vi "Finish.vi"   [LabVIEW 2015]
doc: "This VI is called just before exiting. It is expected to close I/O refnum, save collected data, etc."
uses:
  <vilib>/Rock Robotics/WPI/Utilities/WPI_GetSetVariantRefNum.vi
types:
  T1 = typedef "WPI_DigitalInputDevRef.ctl" = cluster{"DevStatus":errorcluster, "DIO Channel":T2}
  T2 = typedef "FPGA_DIOChannel.ctl" = enum8{"DIO 0", "DIO 1", "DIO 2", "DIO 3", "DIO 4", "DIO 5", "DIO 6", "DIO 7", "DIO 8", "DIO 9", "DIO MXP 0", "DIO MXP 1", "DIO MXP 2", "DIO MXP 3", "DIO MXP 4", "DIO MXP 5", "DIO MXP 6", "DIO MXP 7", "DIO MXP 8", "DIO MXP 9", "DIO MXP 10", "DIO MXP 11", "DIO MXP 12", "DIO MXP 13", "DIO MXP 14", "DIO MXP 15", "Invalid"}
  T3 = typedef "WPI_AccelerometerDevRef.ctl" = cluster{"DevStatus":errorcluster, "Scaling":T4, "Analog Channels":T5, "I2C Bus":T7, "SPI Bus":T8, "Accel Range":T9, "ADXL Axes":T10, "Handle":i32, "Device Address":u8, "Accel Type":enum16{"Analog", "ADXL345 I2C", "ADXL345 SPI", "Internal", "ADXL362 SPI"}}
  T4 = typedef "WPI_AccelerometerScaling.ctl" = cluster{"Gain (VoltsPerG)":dbl, "Center Voltage":dbl}
  T5 = typedef "WPI_AccelerometerAnalogChannels.ctl" = cluster{"X-Axis":T6, "Y-Axis":T6, "Z-Axis":T6}
  T6 = typedef "FPGA_AIChannel.ctl" = enum8{"AI 0", "AI 1", "AI 2", "AI 3", "AI MXP 0", "AI MXP 1", "AI MXP 2", "AI MXP 3", "Invalid"}
  T7 = typedef "i2c_bus.ctl" = enum16{"I2C On-Board", "I2C MXP", "Invalid"}
  T8 = typedef "spi_bus.ctl" = enum16{"SPI On-Board, CS0", "SPI On-Board, CS1", "SPI On-Board, CS2", "SPI On-Board, CS3", "SPI MXP", "Invalid"}
  T9 = typedef "ADXL345 Range.ctl" = u8
  T10 = typedef "WPI_AccelerometerADXL345 Axes.ctl" = cluster{"X-Axis":bool, "Y-Axis":bool, "Z-Axis":bool}
  T11 = typedef "WPI_SolenoidDevRef.ctl" = cluster{"DevStatus":errorcluster, "Pneumatics Control Module":u8, "Forward Solenoid Channel":T12, "Reverse Solenoid Channel":T12}
  T12 = typedef "WPI_SolenoidChannel.ctl" = enum8{"Solenoid 0", "Solenoid 1", "Solenoid 2", "Solenoid 3", "Solenoid 4", "Solenoid 5", "Solenoid 6", "Solenoid 7", "Invalid"}
  T13 = typedef "WPI_ServoDeviceRef.ctl" = cluster{"DeviceStatus":errorcluster, "PWM Channel":T14, "DeadBand":T15}
  T14 = typedef "FPGA_DIOPWMChannel.ctl" = enum8{"PWM 0", "PWM 1", "PWM 2", "PWM 3", "PWM 4", "PWM 5", "PWM 6", "PWM 7", "PWM 8", "PWM 9", "PWM MXP 0", "PWM MXP 1", "PWM MXP 2", "PWM MXP 3", "PWM MXP 4", "PWM MXP 5", "PWM MXP 6", "PWM MXP 7", "PWM MXP 8", "PWM MXP 9", "Invalid"}
  T15 = typedef "WPI_PWMDeadband.ctl" = cluster{"Name":string, "maxPositivePwm":i32, "minPositivePwm":i32, "centerPwm":i32, "maxNegativePwm":i32, "minNegativePwm":i32, "angularRange":u16}
  T16 = typedef "WPI_MotorControlDeviceRef.ctl" = cluster{"DeviceStatus":errorcluster, "Type":T17, "PWM":cluster{"PWM Channel":T14, "DeadBand":T15}, "CAN":cluster{"Device Number":u8, "Control Mode":T18, "Semaphore":T19, "Max Vout":dbl, "TalonSRX Control Mode":T20}, "Invert":bool}
  T17 = typedef "WPI_MotorControlType.ctl" = enum16{"PWM", "CAN", "CANTalonSRX"}
  T18 = typedef "WPI_CANJaguar_ControlMode.ctl" = enum8{"Percent VBus", "Current", "Speed", "Position", "Voltage"}
  T19 = typedef "Semaphore RefNum" = refnum<k1>
  T20 = typedef "WPI_CANTalonSRX_APIControlMode.ctl" = enum8{"Percent VBus", "Speed", "Position", "Slave", "Unchanged / Invalid", "Voltage Compensation", "Current", "Motion Profile"}
  T21 = typedef "WPI_JoystickDevRef.ctl" = cluster{"Device":T22}
  T22 = typedef "WPI_JoystickDeviceEnum.ctl" = enum16{"USB 0", "USB 1", "USB 2", "USB 3", "USB 4", "USB 5"}
  T23 = typedef "WPI_RobotDriveDevRef.ctl" = cluster{"DevStatus":errorcluster, "Motors[]":T16[], "Square Inputs":bool, "Max Output":dbl}
  T24 = typedef "WPI_GyroDevRef.ctl" = cluster{"DevStatus":errorcluster, "Analog Channel":T6, "Offset":dbl, "Gain (VoltsPerDegree/Second)":dbl, "Gyro Type":enum16{"Analog", "XRS450"}, "Handle":i32, "SPI Bus":T8, "Device Found":bool, "Sample Rate":dbl, "Calibrate On Open":bool}
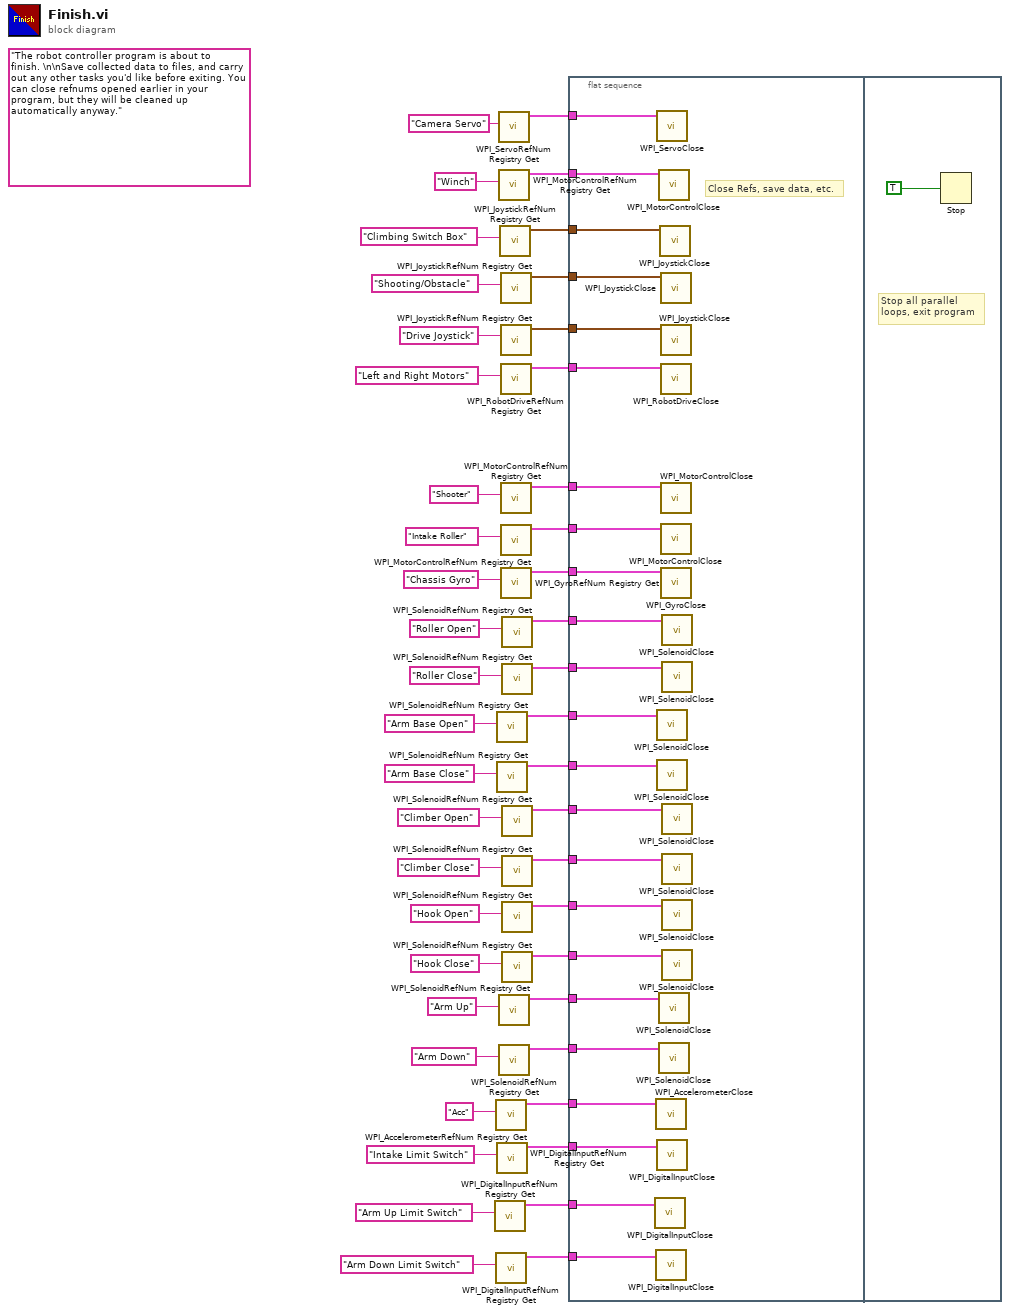
[diagram p0: block diagram]
diagram:
  (unwired) "The robot controller program is about to finish. \n\nSave collected data to files, and carry out any other tasks you'd like before exiting. You can close refnums opened earlier in your program, but they will be cleaned up automatically anyway."
  n1 = call <vilib>:"WPI_DigitalInputRefNum Registry Get.vi"("refnum name"="Arm Up Limit Switch") -> ("DigitalInputDevRef"=w15:T1)  [unwired: 9 in, 1 out]
  n2 = call <vilib>:"WPI_AccelerometerRefNum Registry Get.vi"("refnum name"="Acc") -> ("AccelerometerDevRef"=w36:T3)  [unwired: 9 in, 1 out]
  n3 = call <vilib>:"WPI_DigitalInputRefNum Registry Get.vi"("refnum name"="Arm Down Limit Switch") -> ("DigitalInputDevRef"=w14:T1)  [unwired: 9 in, 1 out]
  n4 = call <vilib>:"WPI_SolenoidRefNum Registry Get.vi"("refnum name"="Arm Base Open") -> ("SolenoidDevRef"=w12:T11)  [unwired: 9 in, 1 out]
  n5 = call <vilib>:"WPI_SolenoidRefNum Registry Get.vi"("refnum name"="Arm Base Close") -> ("SolenoidDevRef"=w9:T11)  [unwired: 9 in, 1 out]
  n6 = call <vilib>:"WPI_DigitalInputRefNum Registry Get.vi"("refnum name"="Intake Limit Switch") -> ("DigitalInputDevRef"=w38:T1)  [unwired: 9 in, 1 out]
  n7 = call <vilib>:"WPI_ServoRefNum Registry Get.vi"("refnum name"="Camera Servo") -> ("ServoDeviceRef"=w2:T13)  [unwired: 9 in, 1 out]
  n8 = call <vilib>:"WPI_MotorControlRefNum Registry Get.vi"("refnum name"="Winch") -> ("MotorControlDevRef"=w17:T16)  [unwired: 9 in, 1 out]
  n9 = call <vilib>:"WPI_SolenoidRefNum Registry Get.vi"("refnum name"="Arm Up") -> ("SolenoidDevRef"=w5:T11)  [unwired: 9 in, 1 out]
  n10 = call <vilib>:"WPI_SolenoidRefNum Registry Get.vi"("refnum name"="Arm Down") -> ("SolenoidDevRef"=w8:T11)  [unwired: 9 in, 1 out]
  n11 = call <vilib>:"WPI_JoystickRefNum Registry Get.vi"("refnum name"="Climbing Switch Box") -> ("JoystickDevRef"=w4:T21)  [unwired: 1 in, 9 out]
  n12 = call <vilib>:"WPI_JoystickRefNum Registry Get.vi"("refnum name"="Shooting/Obstacle") -> ("JoystickDevRef"=w43:T21)  [unwired: 1 in, 9 out]
  n13 = call <vilib>:"WPI_JoystickRefNum Registry Get.vi"("refnum name"="Drive Joystick") -> ("JoystickDevRef"=w32:T21)  [unwired: 1 in, 9 out]
  n14 = call <vilib>:"WPI_RobotDriveRefNum Registry Get.vi"("refnum name"="Left and Right Motors") -> ("RobotDriveDevRef"=w44:T23)  [unwired: 1 in, 9 out]
  n15 = call <vilib>:"WPI_MotorControlRefNum Registry Get.vi"("refnum name"="Shooter") -> ("MotorControlDevRef"=w42:T16)  [unwired: 9 in, 1 out]
  n16 = call <vilib>:"WPI_MotorControlRefNum Registry Get.vi"("refnum name"="Intake Roller") -> ("MotorControlDevRef"=w33:T16)  [unwired: 9 in, 1 out]
  n17 = call <vilib>:"WPI_GyroRefNum Registry Get.vi"("refnum name"="Chassis Gyro") -> ("GyroDevRef"=w40:T24)  [unwired: 9 in, 1 out]
  n18 = call <vilib>:"WPI_SolenoidRefNum Registry Get.vi"("refnum name"="Roller Open") -> ("SolenoidDevRef"=w30:T11)  [unwired: 9 in, 1 out]
  n19 = call <vilib>:"WPI_SolenoidRefNum Registry Get.vi"("refnum name"="Roller Close") -> ("SolenoidDevRef"=w27:T11)  [unwired: 9 in, 1 out]
  n20 = call <vilib>:"WPI_SolenoidRefNum Registry Get.vi"("refnum name"="Climber Open") -> ("SolenoidDevRef"=w23:T11)  [unwired: 9 in, 1 out]
  n21 = call <vilib>:"WPI_SolenoidRefNum Registry Get.vi"("refnum name"="Climber Close") -> ("SolenoidDevRef"=w26:T11)  [unwired: 9 in, 1 out]
  n22 = call <vilib>:"WPI_SolenoidRefNum Registry Get.vi"("refnum name"="Hook Open") -> ("SolenoidDevRef"=w22:T11)  [unwired: 9 in, 1 out]
  n23 = call <vilib>:"WPI_SolenoidRefNum Registry Get.vi"("refnum name"="Hook Close") -> ("SolenoidDevRef"=w19:T11)  [unwired: 9 in, 1 out]
  n24 = flat-sequence {
    tunnel: w44 -> [w69]
    tunnel: w43 -> [w68]
    tunnel: w42 -> [w67]
    tunnel: w40 -> [w66]
    tunnel: w38 -> [w65]
    tunnel: w36 -> [w64]
    tunnel: w33 -> [w63]
    tunnel: w32 -> [w62]
    tunnel: w30 -> [w61]
    tunnel: w27 -> [w60]
    tunnel: w23 -> [w58]
    tunnel: w26 -> [w59]
    tunnel: w22 -> [w57]
    tunnel: w19 -> [w56]
    tunnel: w17 -> [w55]
    tunnel: w15 -> [w54]
    tunnel: w14 -> [w53]
    tunnel: w12 -> [w52]
    tunnel: w9 -> [w51]
    tunnel: w5 -> [w49]
    tunnel: w8 -> [w50]
    tunnel: w4 -> [w48]
    tunnel: w2 -> [w47]
    frame #0 {
      # "Close Refs, save data, etc."
      n25 = call <vilib>:"WPI_DigitalInputClose.vi"("DigitalInputDevRef"=w54) -> ()  [unwired: 10 in, 1 out]
      n26 = call <vilib>:"WPI_AccelerometerClose.vi"("AccelerometerDevRef"=w64) -> ()  [unwired: 10 in, 1 out]
      n27 = call <vilib>:"WPI_DigitalInputClose.vi"("DigitalInputDevRef"=w53) -> ()  [unwired: 10 in, 1 out]
      n28 = call <vilib>:"WPI_ServoClose.vi"("ServoDeviceRef"=w47) -> ()  [unwired: 10 in, 1 out]
      n29 = call <vilib>:"WPI_SolenoidClose.vi"("SolenoidDevRef"=w52) -> ()  [unwired: 10 in, 1 out]
      n30 = call <vilib>:"WPI_SolenoidClose.vi"("SolenoidDevRef"=w51) -> ()  [unwired: 10 in, 1 out]
      n31 = call <vilib>:"WPI_DigitalInputClose.vi"("DigitalInputDevRef"=w65) -> ()  [unwired: 10 in, 1 out]
      n32 = call <vilib>:"WPI_MotorControlClose.vi"("MotorControlDevRef"=w55) -> ()  [unwired: 10 in, 1 out]
      n33 = call <vilib>:"WPI_SolenoidClose.vi"("SolenoidDevRef"=w49) -> ()  [unwired: 10 in, 1 out]
      n34 = call <vilib>:"WPI_SolenoidClose.vi"("SolenoidDevRef"=w50) -> ()  [unwired: 10 in, 1 out]
      n35 = call <vilib>:"WPI_JoystickClose.vi"("JoystickDevRef"=w48) -> ()  [unwired: 11 out]
      n36 = call <vilib>:"WPI_JoystickClose.vi"("JoystickDevRef"=w68) -> ()  [unwired: 11 out]
      n37 = call <vilib>:"WPI_JoystickClose.vi"("JoystickDevRef"=w62) -> ()  [unwired: 11 out]
      n38 = call <vilib>:"WPI_RobotDriveClose.vi"("RobotDriveDevRef"=w69) -> ()  [unwired: 1 in, 10 out]
      n39 = call <vilib>:"WPI_MotorControlClose.vi"("MotorControlDevRef"=w67) -> ()  [unwired: 10 in, 1 out]
      n40 = call <vilib>:"WPI_MotorControlClose.vi"("MotorControlDevRef"=w63) -> ()  [unwired: 10 in, 1 out]
      n41 = call <vilib>:"WPI_GyroClose.vi"("GyroDevRef"=w66) -> ()  [unwired: 10 in, 1 out]
      n42 = call <vilib>:"WPI_SolenoidClose.vi"("SolenoidDevRef"=w61) -> ()  [unwired: 10 in, 1 out]
      n43 = call <vilib>:"WPI_SolenoidClose.vi"("SolenoidDevRef"=w60) -> ()  [unwired: 10 in, 1 out]
      n44 = call <vilib>:"WPI_SolenoidClose.vi"("SolenoidDevRef"=w58) -> ()  [unwired: 10 in, 1 out]
      n45 = call <vilib>:"WPI_SolenoidClose.vi"("SolenoidDevRef"=w59) -> ()  [unwired: 10 in, 1 out]
      n46 = call <vilib>:"WPI_SolenoidClose.vi"("SolenoidDevRef"=w57) -> ()  [unwired: 10 in, 1 out]
      n47 = call <vilib>:"WPI_SolenoidClose.vi"("SolenoidDevRef"=w56) -> ()  [unwired: 10 in, 1 out]
    }
    frame #1 {
      # "Stop all parallel\nloops, exit program"
      n48 = Stop(stop? (T)=TRUE ("Quit")) -> ()
    }
  }
